vi "Waveform Time to second String.vi"(1 "t0":timestamp) -> (0 "String":string)   [LabVIEW 2011]
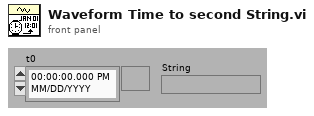
[diagram p1: front panel]
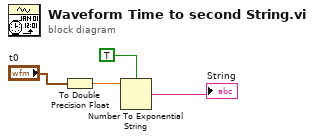
[diagram p0: block diagram]
diagram:
  n1 = To Double Precision Float(number="t0") -> (double precision float=w2:dbl)
  n2 = Number To Exponential String(number=w2, 1:TRUE ("use system decimal point (T)")) -> (E-format string=→"String":string)  [unwired: 2 in]
